vi "Ringdowns.vi"() -> ()   [LabVIEW 2012]
uses:
  Interface/CRDS/Controls/Ringdown Xctl/Ringdown.xctl
  CRDS/Data/cCRDS Data.lvclass
  Reusable/CRDS/Data/Main/Read CellData.vi
  Reusable/CRDS/Data/Cell/CRDS Cell Data.lvclass
panel:
  out "Ringdown":i16[][][](xcontrol)
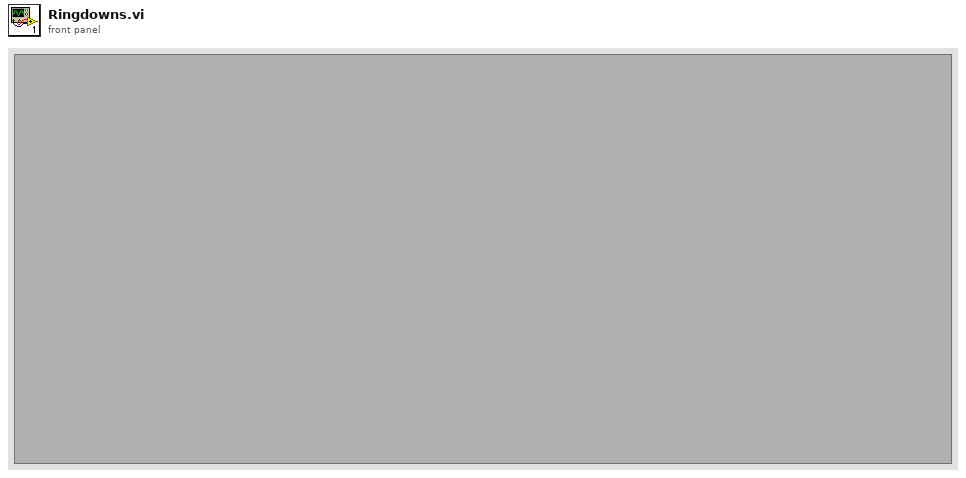
[diagram p1: front panel]
types:
  T1 = cluster{"Read Access":enum8{"Allowed", "Required", "None"}, "Write Access":enum8{"Allowed", "Required", "None"}}
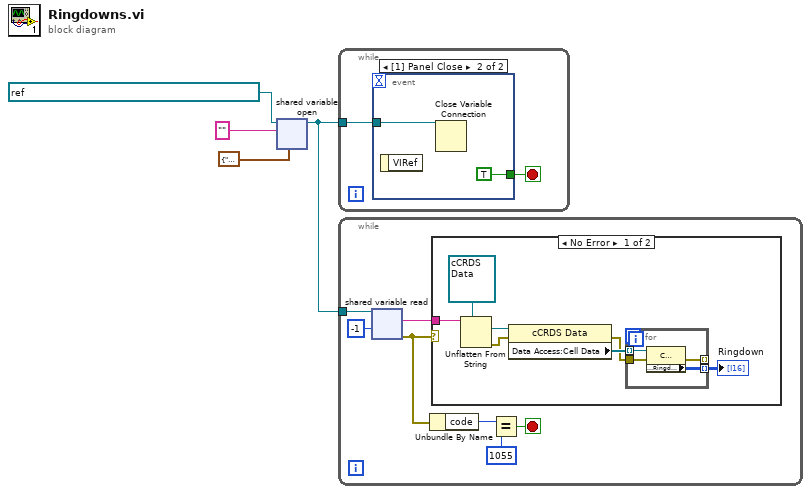
[diagram p0: block diagram]
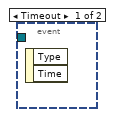
[diagram p3: hidden frame]
diagram:
  n1 = shared-variable-open(refnum<k21> "ni.var.psp://rt pxi target/CRDS_Server/data" ("shared variable refnum in"), "", T1 {"Read Access"=enum."Allowed", "Write Access"=enum."None"} ("access")) -> (w1:refnum<k21>)  [unwired: 1 in, 1 out]
  n2 = while {
    tunnel: w1 -> [w6]
    stop <- w5 stop-if-true
    n3 = event shown="[1] Panel Close" {
      selector: _ -> [_ _]
      dyn-events: _ -> [_ _]
      timeout: _ -> [_ _]
      tunnel: w6 -> [_ w8]
      tunnel: [_ TRUE] -> w5
      event Timeout {
        n4 = event-data() -> ()  [unwired: 1 in, 2 out]
      }
      event Panel Close {
        n5 = event-data() -> ()  [unwired: 1 in, 1 out]
        n6 = Close Variable Connection(11:w8) -> ()  [unwired: 1 in, 1 out]
      }
    }
  }
  n7 = while {
    tunnel: w1 -> [w15]
    stop <- w10 stop-if-true
    n8 = shared-variable-read(w15, -1 ("timeout ms")) -> (w11:errorcluster, w14:string)  [unwired: 1 in, 3 out]
    n9 = Unbundle By Name(w11) -> ("code"=w13:i32)
    n10 = case shown="No Error" w11 {
      tunnel: w14 -> [w21 _]
      frame No Error {
        n11 = Unflatten From String(type=refnum<class "cCRDS Data.lvclass"> refnum ("cCRDS Data"), binary string=w21) -> (value=w20:refnum<class "cCRDS Data.lvclass">, error out=w19:errorcluster)  [unwired: 3 in, 1 out]
        n12 = property class="cCRDS Data"(reference=w20, error in=w19) -> (error out=w17:errorcluster, "Data Access:Cell Data"=w18:refnum<class "CRDS Cell Data.lvclass">[])  [unwired: 1 out]
        n13 = for {
          tunnel: w18 -> [w26] mode=indexing
          tunnel: [w25] -> w16 mode=indexing
          tunnel: [w24] -> _ mode=indexing
          tunnel: w17 -> [w23]
          n14 = property class="CRDS Cell"(reference=w26, error in=w23) -> (error out=w24:errorcluster, "Data Access:Ringdowns"=w25:i16[][])  [unwired: 1 out]
        }
        "Ringdown" <- w16
      }
      frame Error {
      }
    }
    n15 = Equal?(x=w13, y=1055) -> (x = y?=w10:bool)
  }
